vi "Cmd Get Command Properties (CR).vi"(4 "error in (no error)":errorcluster, 7 "command-recordset reference":T2) -> (0 "error out":errorcluster, 1 "command properties":T1, 3 "command-recordset reference out":T2)   [LabVIEW 2012, in "NI_Database_API_64.lvlib"]
doc: "Gets properties of the object as determined by the inputs. This VI works for connections, commands, recordsets, columns, and parameters. Wire data to the reference input to determine the polymorphic instance to use or manually select the instance."
uses:
  NI_Database_API_64.lvlib
  Command-Recordset.llb/Cmd-Rec Object Reference.ctl
  Cmd Properties.ctl
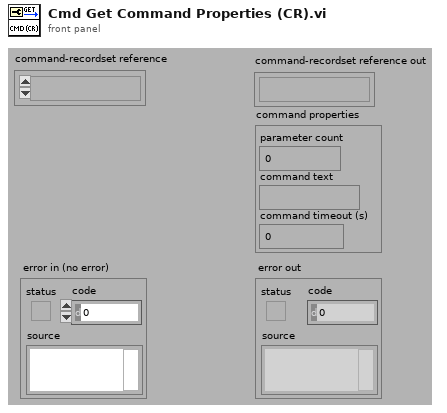
[diagram p1: front panel]
types:
  T1 = typedef "NI_Database_API_64.lvlib/Cmd Properties.ctl" = cluster{"parameter count":i32, "command text":string, "command timeout (s)":i32}
  T2 = typedef "NI_Database_API_64.lvlib/Cmd-Rec Object Reference.ctl" = refnum<k1>
  T3 = typedef "NI_Database_API_64.lvlib/Cmd-Rec Data Members.ctl" = cluster{"recordset reference":T4, "command reference":T5}
  T4 = typedef "NI_Database_API_64.lvlib/Rec ObjectReference.ctl" = refnum<k1>
  T5 = typedef "NI_Database_API_64.lvlib/Cmd ObjectReference.ctl" = refnum<k1>
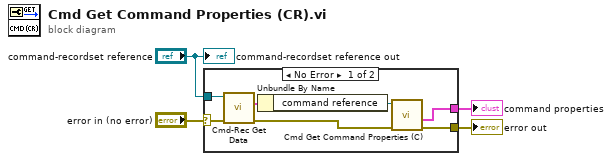
[diagram p0: block diagram]
diagram:
  n1 = case shown="No Error" "error in (no error)" {
    selector: "error in (no error)" -> [w5 w12]
    tunnel: [w11 w12] -> w4
    tunnel: [w10 _] -> w3
    tunnel: "command-recordset reference" -> [w7 _]
    frame No Error {
      n2 = call "Cmd-Rec Get Data.vi"("error in (no error)"=w5, "command-recordset reference"=w7) -> ("error out"=w6:errorcluster, "data"=w8:T3)  [unwired: 2 in, 2 out]
      n3 = Unbundle By Name(w8) -> ("command reference"=w9:T5)
      n4 = call "Cmd Get Command Properties (C).vi"("error in (no error)"=w6, "command reference"=w9) -> ("error out"=w11:errorcluster, "command properties"=w10:T1)  [unwired: 3 in, 1 out]
    }
    frame Error {
    }
  }
  "error out" <- w4
  "command properties" <- w3
  "command-recordset reference out" <- "command-recordset reference"
